vi "Broken Springs Block Math.vi"(9 "index":u8, 11 "contiguous length of broken springs":u8[](array[numeric])) -> (1 "right total":u8, 2 "current index broken streak length":u8, 3 "left total":u8)   [LabVIEW 2022 SP3]
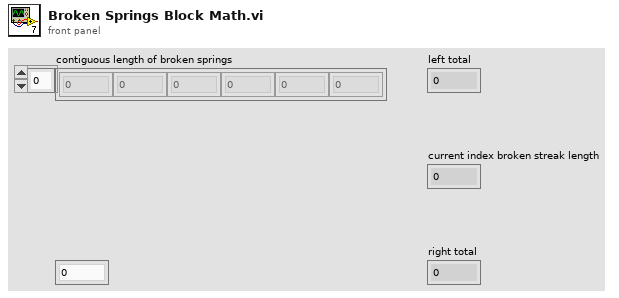
[diagram p1: front panel]
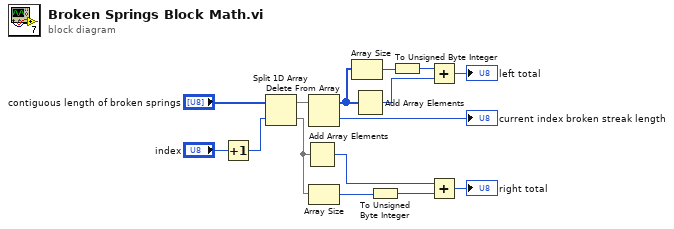
[diagram p0: block diagram]
diagram:
  n1 = Increment(x="index") -> (x+1=w5:u8)
  n2 = Split 1D Array(array="contiguous length of broken springs", index=w5) -> (first subarray=w11:u8[], second subarray=w7:u8[])
  n3 = Add Array Elements(numeric array=w7) -> (sum=w8:u8)
  n4 = Delete From Array(array=w11) -> (deleted portion=→"current index broken streak length":u8, array with subset deleted=w3:u8[])  [unwired: 2 in]
  n5 = Array Size(array=w7) -> (size(s)=w9:i32)
  n6 = Array Size(array=w3) -> (size(s)=w10:i32)
  n7 = Add Array Elements(numeric array=w3) -> (sum=w12:u8)
  n8 = To Unsigned Byte Integer(number=w9) -> (unsigned 8bit integer=w1:u8)
  n9 = To Unsigned Byte Integer(number=w10) -> (unsigned 8bit integer=w2:u8)
  n10 = Add(x=w2, y=w12) -> (x+y=→"left total":u8)
  n11 = Add(x=w8, y=w1) -> (x+y=→"right total":u8)
